vi "Determine if name or container.vi"(8 "error in (no error)":errorcluster, 11 "Name or Namespace":string) -> (0 "error out":errorcluster, 3 "Is Container?":bool)   [LabVIEW 2018, in "Path and String Processing.lvlib"]
uses:
  Path and String Processing.lvlib
  <vilib>/regexp/Match Regular Expression.xnode
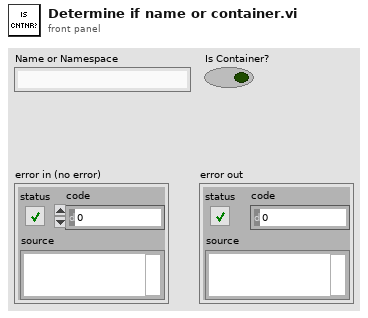
[diagram p1: front panel]
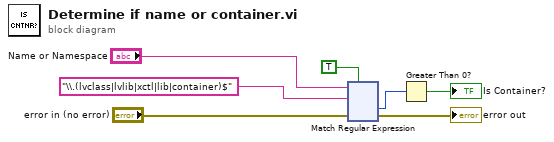
[diagram p0: block diagram]
diagram:
  n1 = xnode "Match Regular Expression"("input string"="Name or Namespace", "regular expression"="\\.(lvclass|lvlib|xctl|lib|container)$", "error in"="error in (no error)", "ignore case? (F)"=TRUE) -> ("offset past match"=w3:i32, "error out"=→"error out":errorcluster)  [unwired: 2 in, 3 out]
  n2 = Greater Than 0?(x=w3) -> (x > 0?=→"Is Container?":bool)
